vi "Process.vi"(9 "Module Info In":T1, 11 "Engine Tags In":T3) -> (1 "Module Info Out":T1, 3 "Engine Tags Out":T3)   [LabVIEW 2013, in "Standard Engine Runtime.lvclass"]
uses:
  Standard Engine Runtime.lvclass
  <vilib>/NI/Tag Bus/table/data table.ctl
  Module Execution Info.ctl
  <vilib>/NI/Tag Bus Module Framework/runtime/TBM module execution interface.lvclass
  Data Table with Transfer Spec.ctl
  <vilib>/NI/Tag Bus/table/transfer specification.ctl
  <vilib>/NI/Tag Bus/tag/Data Type.ctl
  Configuration/Module Decimation.ctl
  Configuration/Module Error Configuration.ctl
  Configuration/Error Actions By Category.ctl
  <vilib>/NI/Tag Bus Module Framework/runtime/error classification.ctl
  Configuration/Error Actions.ctl
  <vilib>/NI/Tag Bus/table/data table.lvlib
  <vilib>/NI/Tag Bus/tag/tag descriptor.lvclass
  Configuration/Standard Engine Configuration.lvclass
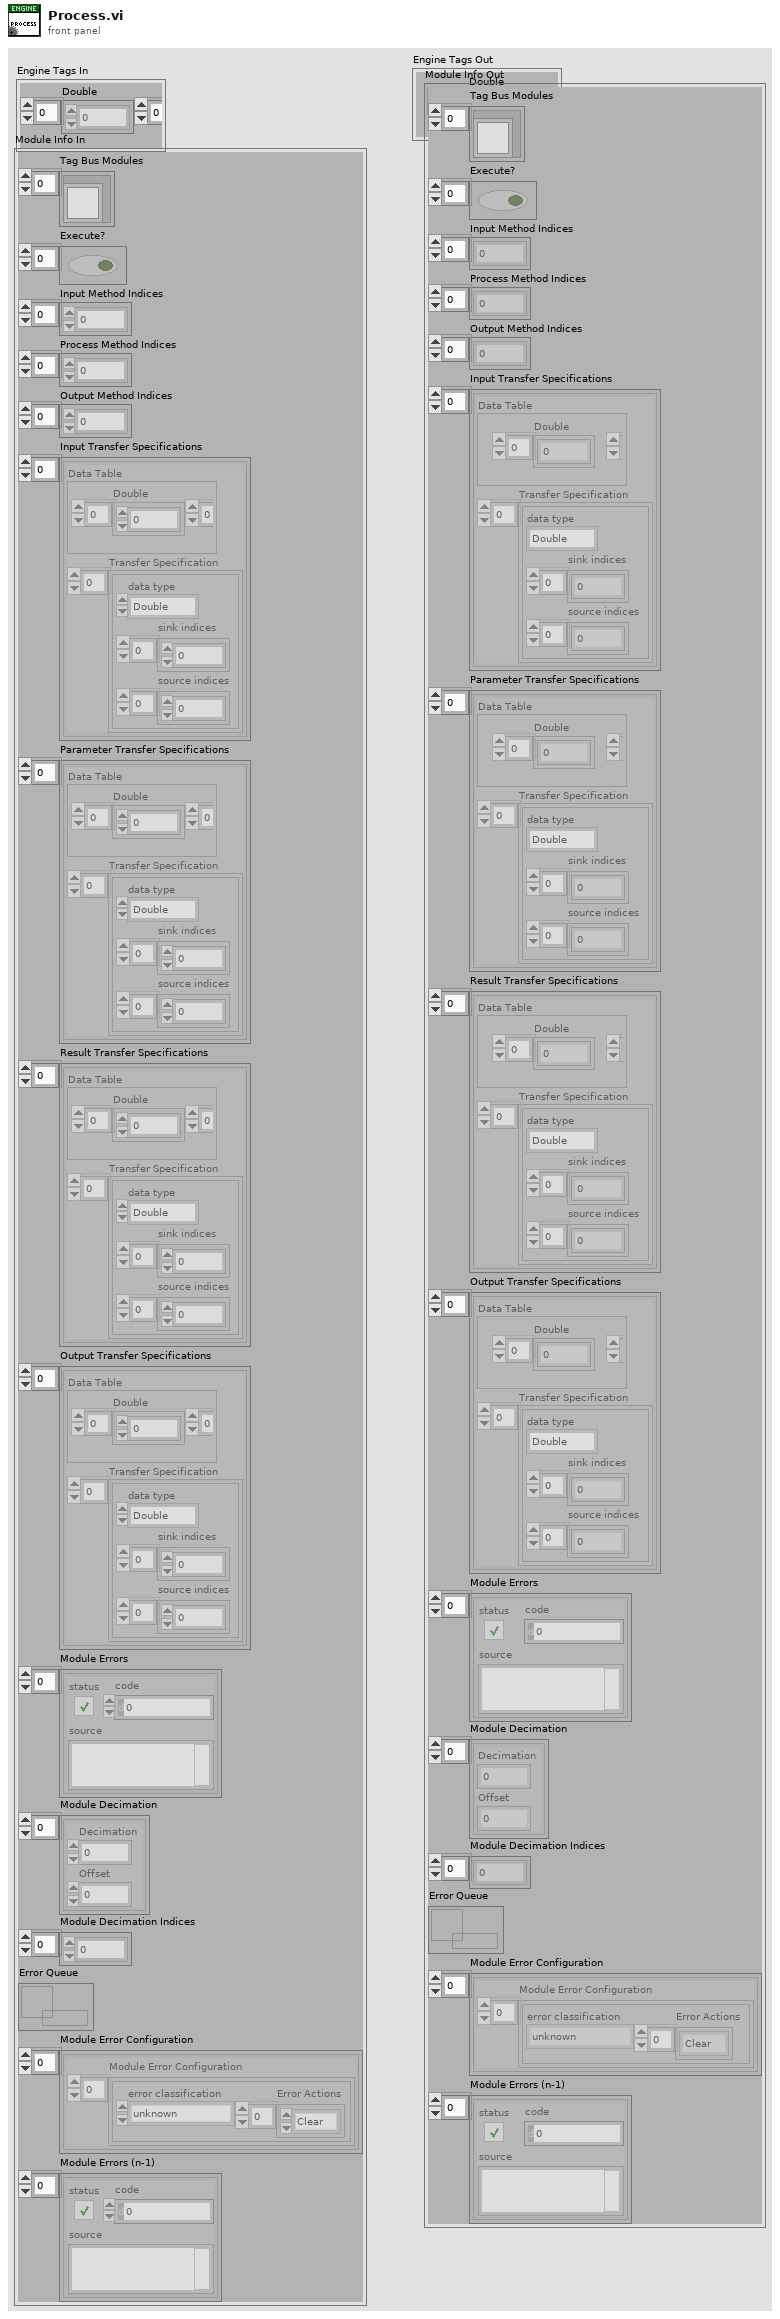
[diagram p1: front panel]
types:
  T1 = typedef "Standard Engine Runtime.lvclass/Module Execution Info.ctl" = cluster{"Tag Bus Modules":refnum<class "TBM module execution interface.lvclass">[], "Execute?":bool[], "Input Method Indices":i32[], "Process Method Indices":i32[], "Output Method Indices":i32[], "Input Transfer Specifications":T2[], "Parameter Transfer Specifications":T2[], "Result Transfer Specifications":T2[], "Output Transfer Specifications":T2[], "Module Errors":errorcluster[], "Module Decimation":T6[], "Module Decimation Indices":i32[], "Error Queue":refnum<queue>, "Module Error Configuration":T7[], "Module Errors (n-1)":errorcluster[]}
  T2 = typedef "Standard Engine Runtime.lvclass/Data Table with Transfer Spec.ctl" = cluster{"Data Table":T3, "Transfer Specification":T4[]}
  T3 = typedef "tag bus.lvlib/data table.lvlib/data table.ctl" = cluster{"Double":dbl[], "Single":sgl[], "I64":i64[], "I32":i32[], "I16":i16[], "I8":i8[], "U64":u64[], "U32":u32[], "U16":u16[], "U8":u8[], "Boolean":bool[], "String":string[], "Array of Double":cluster{"DBL Array":dbl[]}[], "Array of Single":cluster{"SGL Array":sgl[]}[], "Array of I64":cluster{"I64 Array":i64[]}[], "Array of I32":cluster{"I32 Array":i32[]}[], "Array of I16":cluster{"I16 Array":i16[]}[], "Array of I8":cluster{"I8 Array":i8[]}[], "Array of U64":cluster{"U64 Array":u64[]}[], "Array of U32":cluster{"U32 Array":u32[]}[], "Array of U16":cluster{"U16 Array":u16[]}[], "Array of U8":cluster{"U8 Array":u8[]}[], "Array of Boolean":cluster{"Boolean Array":bool[]}[], "Array of String":cluster{"String Array":string[]}[]}
  T4 = typedef "tag bus.lvlib/data table.lvlib/transfer specification.ctl" = cluster{"data type":T5, "sink indices":i32[], "source indices":i32[]}
  T5 = typedef "tag bus.lvlib/tag descriptor.lvclass/Data Type.ctl" = enum16{"Double", "Single", "I64", "I32", "I16", "I8", "U64", "U32", "U16", "U8", "Boolean", "String", "Array of Double", "Array of Single", "Array of I64", "Array of I32", "Array of I16", "Array of I8", "Array of U64", "Array of U32", "Array of U16", "Array of U8", "Array of Boolean", "Array of String"}
  T6 = typedef "Standard Engine Configuration.lvclass/Module Decimation.ctl" = cluster{"Decimation":u16, "Offset":u16}
  T7 = typedef "Standard Engine Configuration.lvclass/Module Error Configuration.ctl" = cluster{"Module Error Configuration":T8[]}
  T8 = typedef "Standard Engine Configuration.lvclass/Error Actions By Category.ctl" = cluster{"error classification":T9, "Error Actions":T10[]}
  T9 = typedef "TBM module execution interface.lvclass/error classification.ctl" = enum16{"unknown", "none", "trivial", "recoverable", "critical"}
  T10 = typedef "Standard Engine Configuration.lvclass/Error Actions.ctl" = enum16{"Clear", "Notify", "Stop Component", "Stop Engine", "Safe State", "Attempt Recovery"}
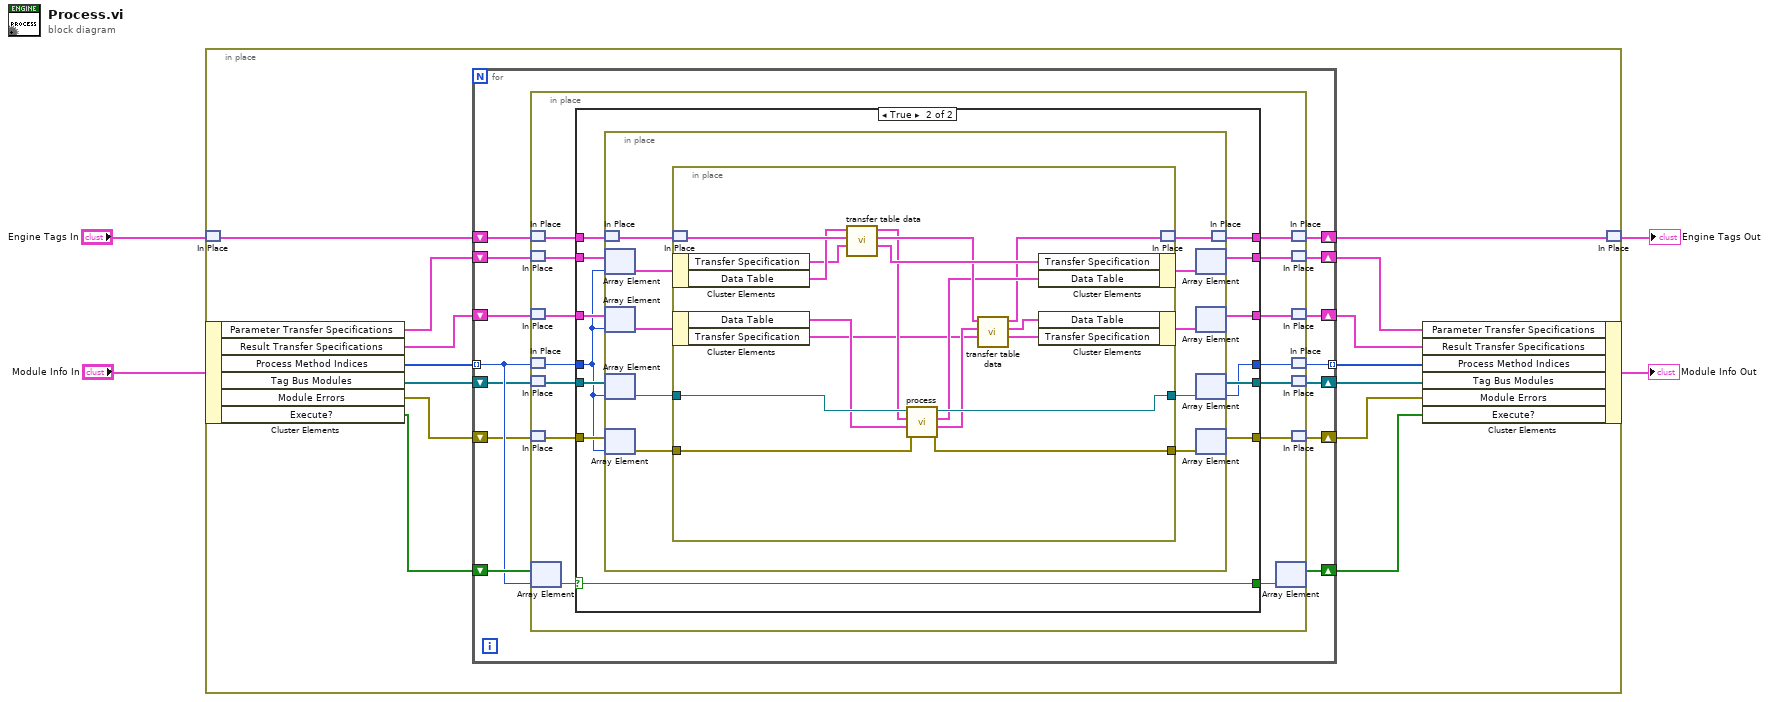
[diagram p0: block diagram]
diagram:
  n1 = in-place {
    n2 = in-place-match #1("Engine Tags In") -> (w18:T3)
    n3 = in-place-cluster #2("Module Info In") -> ("Parameter Transfer Specifications"=w16:T2[], "Result Transfer Specifications"=w13:T2[], "Process Method Indices"=w9:i32[], "Tag Bus Modules"=w10:refnum<class "TBM module execution interface.lvclass">[], "Module Errors"=w15:errorcluster[], "Execute?"=w6:bool[])
    n4 = for {
      shift-right: [w21] -> w7
      shift-left: w10 -> [w22]
      shift-right: [w29] -> w17
      shift-left: w18 -> [w30]
      shift-right: [w27] -> w12
      shift-left: w16 -> [w28]
      shift-right: [w19] -> w14
      shift-left: w15 -> [w20]
      shift-right: [w25] -> w11
      shift-left: w13 -> [w26]
      tunnel: [w23] -> w8 mode=indexing
      tunnel: w9 -> [w24] mode=indexing
      shift-right: [w31] -> w5
      shift-left: w6 -> [w32]
      n5 = in-place {
        n6 = in-place-match #3(w30) -> (w44:T3)
        n7 = in-place-match #4(w28) -> (w42:T2[])
        n8 = in-place-match #5(w26) -> (w40:T2[])
        n9 = in-place-match #6(w24) -> (w38:i32)
        n10 = in-place-match #7(w22) -> (w36:refnum<class "TBM module execution interface.lvclass">[])
        n11 = in-place-match #8(w20) -> (w34:errorcluster[])
        n12 = in-place-array #9(w32, w24) -> (w46:bool)
        n13 = case shown="True" w46 {
          selector: w46 -> [w47 w56]
          tunnel: w44 -> [w53 w66]
          tunnel: [w53 w65] -> w43
          tunnel: w42 -> [w52 w64]
          tunnel: w40 -> [w51 w63]
          tunnel: w36 -> [w49 w62]
          tunnel: w34 -> [w48 w61]
          tunnel: [w48 w60] -> w33
          tunnel: [w49 w59] -> w35
          tunnel: [w52 w58] -> w41
          tunnel: [w51 w57] -> w39
          tunnel: [w50 w55] -> w37
          tunnel: w38 -> [w50 w54]
          tunnel: [w47 w56] -> w45
          frame False {
          }
          frame True {
            n14 = in-place {
              n15 = in-place-match #10(w66) -> (w72:T3)
              n16 = in-place-array #11(w64, w54) -> (w70:T2)
              n17 = in-place-array #12(w63, w54) -> (w69:T2)
              n18 = in-place-array #13(w62, w54) -> (w76:refnum<class "TBM module execution interface.lvclass">)
              n19 = in-place-array #14(w61, w54) -> (w74:errorcluster)
              n20 = in-place {
                in-place-border: w76 -> [w93]
                in-place-border: [w92] -> w75
                in-place-border: w74 -> [w91]
                in-place-border: [w90] -> w73
                n21 = in-place-match #15(w72) -> (w89:T3)
                n22 = in-place-cluster #16(w70) -> ("Transfer Specification"=w87:T4[], "Data Table"=w88:T3)
                n23 = in-place-cluster #17(w69) -> ("Data Table"=w83:T3, "Transfer Specification"=w80:T4[])
                n24 = call <vilib>:"transfer table data.vi"("transfer specification in"=w87, "data table source in"=w89, "data table sink in"=w88) -> ("transfer specification out"=w86:T4[], "data table source out"=w85:T3, "data table sink out"=w84:T3)  [unwired: 6 in]
                n25 = call-dynamic "process.vi"("error in"=w91, "result allocation"=w83, "parameters"=w84, "module in"=w93) -> ("error out"=w90:errorcluster, "results"=w81:T3, "parameter allocation"=w82:T3, "module out"=w92:refnum<class "TBM module execution interface.lvclass">)  [unwired: 4 in]
                n26 = call <vilib>:"transfer table data.vi"("transfer specification in"=w80, "data table source in"=w81, "data table sink in"=w85) -> ("transfer specification out"=w79:T4[], "data table source out"=w78:T3, "data table sink out"=w77:T3)  [unwired: 6 in]
                n27 = in-place-cluster #16("Transfer Specification"=w86, "Data Table"=w82) -> (w67:T2)
                n28 = in-place-cluster #17("Data Table"=w78, "Transfer Specification"=w79) -> (w68:T2)
                n29 = in-place-match #15(w77) -> (w71:T3)
              }
              n30 = in-place-array #11(w67) -> (w58:T2[])  [unwired: 1 out]
              n31 = in-place-array #12(w68) -> (w57:T2[])  [unwired: 1 out]
              n32 = in-place-array #13(w75) -> (w59:refnum<class "TBM module execution interface.lvclass">[], w55:i32)
              n33 = in-place-array #14(w73) -> (w60:errorcluster[])  [unwired: 1 out]
              n34 = in-place-match #10(w71) -> (w65:T3)
            }
          }
        }
        n35 = in-place-array #9(w45) -> (w31:bool[])  [unwired: 1 out]
        n36 = in-place-match #3(w43) -> (w29:T3)
        n37 = in-place-match #4(w41) -> (w27:T2[])
        n38 = in-place-match #5(w39) -> (w25:T2[])
        n39 = in-place-match #6(w37) -> (w23:i32)
        n40 = in-place-match #7(w35) -> (w21:refnum<class "TBM module execution interface.lvclass">[])
        n41 = in-place-match #8(w33) -> (w19:errorcluster[])
      }
    }
    n42 = in-place-cluster #2("Parameter Transfer Specifications"=w12, "Result Transfer Specifications"=w11, "Process Method Indices"=w8, "Tag Bus Modules"=w7, "Module Errors"=w14, "Execute?"=w5) -> (→"Module Info Out":T1)
    n43 = in-place-match #1(w17) -> (→"Engine Tags Out":T3)
  }
